vi "Prefilter_60Hz_Notch.vi"(11 "Array":waveform(dbl)[](array[waveform])) -> (3 "Array 2":waveform(dbl)[](array[waveform]))   [LabVIEW 2016, in "lockin.lvclass"]
uses:
  lockin.lvclass
  <vilib>/addons/Digital Filter Design/Design.llb/DFD IIR Notch Peak Design by Q.vi
  <vilib>/addons/Digital Filter Design/Process.llb/DFD Filtering (Wfm NChan).vi
  <vilib>/addons/Digital Filter Design/NI_DigFilterLicensed.lvlib
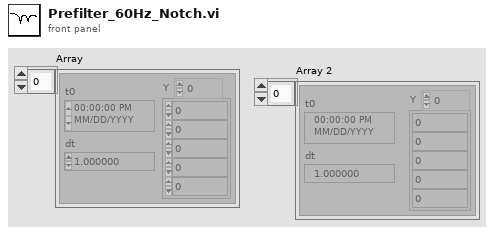
[diagram p1: front panel]
types:
  T1 = typedef "NI_DigFilterLicensed.lvlib/DFD Filter Obj.ctl" = cluster{"mSRate_Fs":dbl, "mSRate_Version":string, "mSRate_Comments":string, "mSRate_OrgCoef":T2, "mSRate_CurCoef":T2, "mSRate_Quantized?":bool, "mSRate_QCoef":T2, "mSRate_QSettings":T4[], "mSRate_Order":i32, "mSRate_Scaling":cluster{"mSRate_ScaleByPowerOf2?":bool, "mSRate_ScaleType":T6}}
  T2 = typedef "NI_DigFilterLicensed.lvlib/DFD Filter Coef.ctl" = cluster{"type":T3, "gain":dbl, "coef a (k)":dbl[], "coef b (v)":dbl[]}
  T3 = typedef "NI_DigFilterLicensed.lvlib/DFD Filter Structure Type Selector.ctl" = enum16{"Undefined", "FIR Direct Form", "FIR Direct Form Transposed", "FIR Symmetric", "FIR Antisymmetric", "IIR Direct Form I", "IIR Direct Form I Transposed", "IIR Direct Form II", "IIR Direct Form II Transposed", "IIR Cascaded Second Order Sections Form I", "IIR Cascaded Second Order Sections Form I Transposed", "IIR Cascaded Second Order Sections Form II", "IIR Cascaded Second Order Sections Form II Transposed", "Lattice Allpass (basic sections)", "Lattice Allpass (one multiplier sections)", "Lattice Allpass (normalized sections)", "Lattice AR (basic sections)", "Lattice AR (one multiplier sections)", "Lattice AR (normalized sections)", "Lattice MA (minimum phase)", "Lattice MA (maximum phase)", "Lattice ARMA (basic sections)", "Lattice ARMA (one multiplier sections)", "Lattice ARMA (normalized sections)"}
  T4 = typedef "NI_DigFilterLicensed.lvlib/dfd_Internal Quantization Settings.ctl" = cluster{"source":T5, "wl":i16, "iwl":i16, "overflow mode":enum16{"Saturation", "Wrap"}, "rounding mode":enum16{"Nearest", "Truncation"}, "signed?":bool}
  T5 = typedef "NI_DigFilterLicensed.lvlib/dfd_Internal Quantization Srcs.ctl" = u16
  T6 = typedef "NI_DigFilterLicensed.lvlib/DFD Coef Norm Type.ctl" = enum16{"No Norm", "Time Domain 1-Norm", "Time Domain 2-Norm", "Time Domain Inf-Norm"}
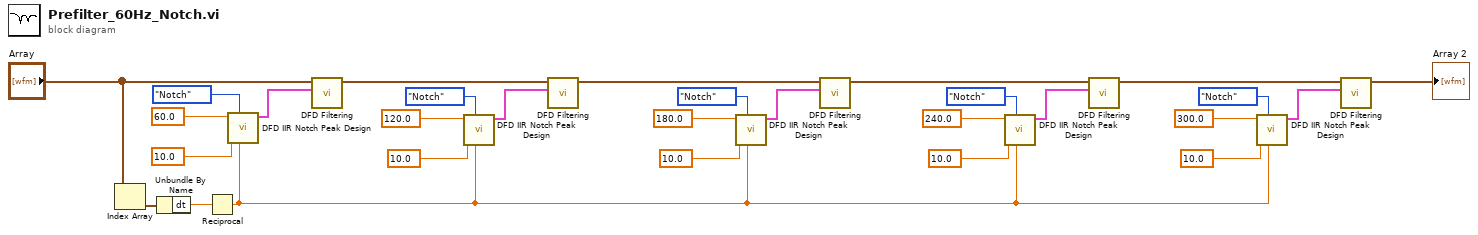
[diagram p0: block diagram]
diagram:
  n1 = Index Array(array="Array") -> (element=w25:waveform(dbl))  [unwired: 1 in]
  n2 = Unbundle By Name(w25) -> ("dt"=w28:dbl)
  n3 = Reciprocal(x=w28) -> (1/x=w1:dbl)
  n4 = call-poly <vilib>:"DFD IIR Notch Peak Design.vi"("fs [Hz]"=w1, "filter type"=enum16{"Notch", "Peak"}."Notch", "Q factor"=10.0, "f0 [Hz]"=60.0) -> ("filter out"=w27:T1)  [unwired: 6 in, 1 out]
  n5 = call-poly <vilib>:"DFD Filtering.vi"("filter"=w27, "signal in"="Array") -> ("signal out"=w20:waveform(dbl)[])  [unwired: 8 in, 1 out]
  n6 = call-poly <vilib>:"DFD IIR Notch Peak Design.vi"("fs [Hz]"=w1, "filter type"=enum16{"Notch", "Peak"}."Notch", "Q factor"=10.0, "f0 [Hz]"=120.0) -> ("filter out"=w19:T1)  [unwired: 6 in, 1 out]
  n7 = call-poly <vilib>:"DFD Filtering.vi"("filter"=w19, "signal in"=w20) -> ("signal out"=w4:waveform(dbl)[])  [unwired: 8 in, 1 out]
  n8 = call-poly <vilib>:"DFD IIR Notch Peak Design.vi"("fs [Hz]"=w1, "filter type"=enum16{"Notch", "Peak"}."Notch", "Q factor"=10.0, "f0 [Hz]"=180.0) -> ("filter out"=w17:T1)  [unwired: 6 in, 1 out]
  n9 = call-poly <vilib>:"DFD Filtering.vi"("filter"=w17, "signal in"=w4) -> ("signal out"=w3:waveform(dbl)[])  [unwired: 8 in, 1 out]
  n10 = call-poly <vilib>:"DFD IIR Notch Peak Design.vi"("fs [Hz]"=w1, "filter type"=enum16{"Notch", "Peak"}."Notch", "Q factor"=10.0, "f0 [Hz]"=240.0) -> ("filter out"=w10:T1)  [unwired: 6 in, 1 out]
  n11 = call-poly <vilib>:"DFD Filtering.vi"("filter"=w10, "signal in"=w3) -> ("signal out"=w2:waveform(dbl)[])  [unwired: 8 in, 1 out]
  n12 = call-poly <vilib>:"DFD IIR Notch Peak Design.vi"("fs [Hz]"=w1, "filter type"=enum16{"Notch", "Peak"}."Notch", "Q factor"=10.0, "f0 [Hz]"=300.0) -> ("filter out"=w9:T1)  [unwired: 6 in, 1 out]
  n13 = call-poly <vilib>:"DFD Filtering.vi"("filter"=w9, "signal in"=w2) -> ("signal out"=→"Array 2":waveform(dbl)[])  [unwired: 8 in, 1 out]
